vi "CAN BL Write.vi"(4 "TimeOut":u32, 5 "DataNum":u32, 6 "pData":string, 7 "AddrOffset":u32, 9 "NodeAddr":u16, 10 "CANIndex":i32, 11 "DevHandle":i32) -> (2 "function return":i32, 3 "pData out":string)   [LabVIEW 2010, in "usb2can.lvlib"]
doc: "int WINAPI CAN_BL_Write(int DevHandle,int CANIndex,unsigned short NodeAddr,unsigned int AddrOffset,unsigned char *pData,unsigned int DataNum,unsigned int TimeOut);"
uses:
  usb2can.lvlib
  USB2XXX.dll
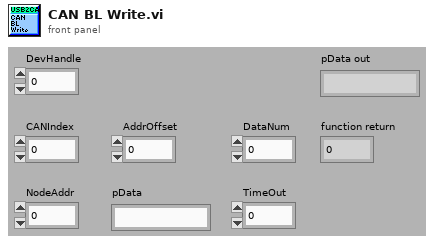
[diagram p1: front panel]
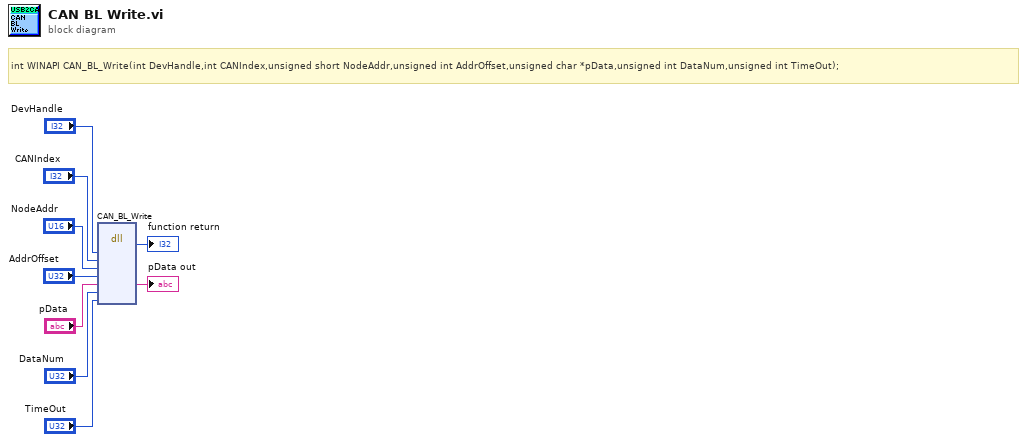
[diagram p0: block diagram]
diagram:
  # "int WINAPI CAN_BL_Write(int DevHandle,int CANIndex,unsigned short NodeAddr,unsigned int AddrOffset,unsigned char *pData,unsigned int DataNum,unsigned int TimeOut);"
  n1 = dll-call lib="E:/OtherWork/STM32/USB2XXX_Example/sdk/api/Labview/USB2XXX.*" fn="CAN_BL_Write"("DevHandle"="DevHandle", "CANIndex"="CANIndex", "NodeAddr"="NodeAddr", "AddrOffset"="AddrOffset", "pData"="pData", "DataNum"="DataNum", "TimeOut"="TimeOut") -> (→"function return":i32, "pData"=→"pData out":string)  [unwired: 9 in, 2 out]
